vi "niScope Configure Acquisition.vi"(0 "instrument handle":refnum<k15>, 7 "acquisition Type":T1 items=["Normal"=0, "Flex Res"=1, "DDC"=3], 11 "error in":errorcluster) -> (4 "instrument handle out":refnum<k15>, 15 "error out":errorcluster)   [LabVIEW 2013]
doc: "Configures how the digitizer acquires data and fills the waveform record."
uses:
  <instrlib>/niScope/Controls/niScope acquisition type.ctl
  niScope_32.dll
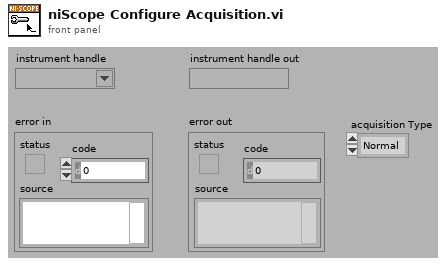
[diagram p1: front panel]
types:
  T1 = typedef "niScope acquisition type.ctl" = i32
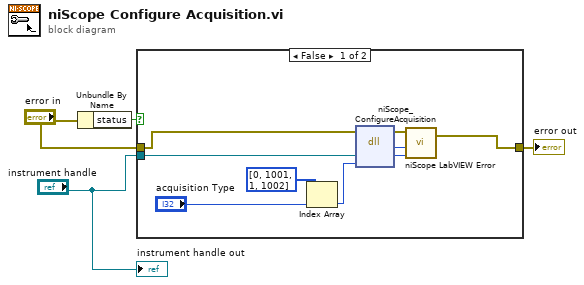
[diagram p0: block diagram]
diagram:
  n1 = Unbundle By Name("error in") -> ("status"=w3:bool)
  n2 = case shown="False" w3 {
    tunnel: "error in" -> [w8 w13]
    tunnel: [w7 w13] -> w2
    tunnel: "instrument handle" -> [w12 _]
    frame False {
      n3 = Index Array(array=i32[] [0, 1001, 1, 1002] ("Array"), index="acquisition Type") -> (element=w11:i32)
      n4 = dll-call lib="niScope_*.*" fn="niScope_ConfigureAcquisition"("instrument handle"=w12, "acquisitionType"=w11) -> ("status"=w10:i32, "instrument handle"=w9:u32)  [unwired: 4 in, 2 out]
      n5 = call <instrlib>:"niScope LabVIEW Error.vi"("instrument handle"=w9, "niScope error code (0)"=w10, "error in (no error)"=w8) -> ("error out"=w7:errorcluster)  [unwired: 2 in]
    }
    frame True {
    }
  }
  "error out" <- w2
  "instrument handle out" <- "instrument handle"
